vi "nifxpmath_DesktopException.vi"() -> ()   [LabVIEW 2017]
panel:
  out "undefined exception":string="LabVIEW FPGA:  An internal software error in the LabVIEW FPGA Module has occurred.  Please contact National Instruments technical support at ni.com/support."
  out "memory full exception":string="Memory is full."
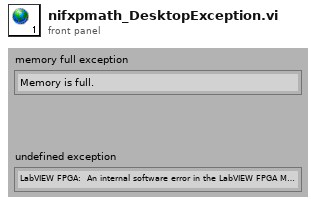
[diagram p1: front panel]
diagram:
